vi "Execute Statement.vi"(8 "error in (no error)":errorcluster, 10 "SQL statement":string, 11 "SQLite3LV Cursor in":refnum<class "cursor.lvclass">) -> (0 "error out":errorcluster, 3 "SQLite3LV Cursor out":refnum<class "cursor.lvclass">)   [LabVIEW 2014, in "SQLite3LV.lvlib" / "cursor.lvclass"]
doc: "Executes a single SQL statement. If multiple statements are included in the SQL statement input, only the first statement will be executed.\n\nThe statement may contain unnamed parameters and may return query results.\n\nExamples:\n\nSELECT `LastName` from `Persons`;\n Returns zero or more results of type string. Use \"Column String\" property, followed by the \"Rows Finished?\" property to retrieve results.\n\nSELECT `LastName` from `Persons` WHERE `LastName` GLOB ?\n Returns zero or more results of type string. One string-typed query parameter. Use the \"Bind String\" property node after executing the query to bind the parameter. Use the \"Column String\" and \"Rows Finished?\" property to retrieve results.\n\nSELECT ? + ?;\n Returns a single result of arbitrary type. Accepts two parameters of arbitrary type. Use the \"Bind DBL\" two bind two input parameters. Use the \"Column DBL\" to retrieve the query result."
uses:
  cursor.lvclass
  cursor.lvclass/cursor.ctl
  SQLite3LV.lvlib
  SQLite3 Class/sqlite3.lvclass
  sqlite3_64.dll
panel:
  out "finished?":bool
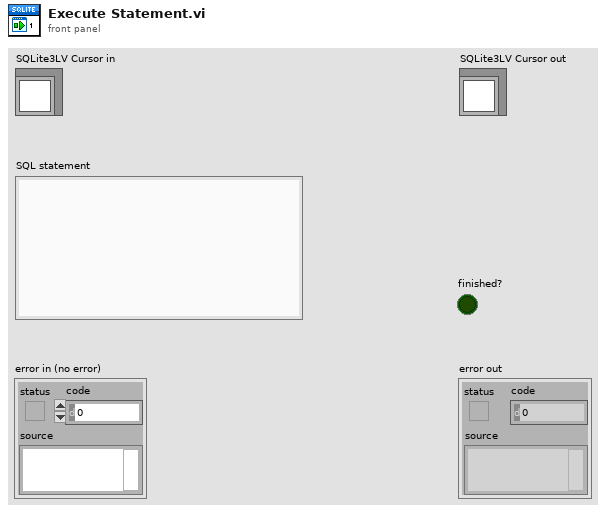
[diagram p1: front panel]
types:
  T1 = typedef "SQLite3LV.lvlib/cursor.lvclass/ctl_active_statement.ctl" = cluster{"ppStmt":i64, "column count":i32, "bind offset":i32, "bind param count":i32, "finished?":bool, "column offset":i32, "column types":i32[]}
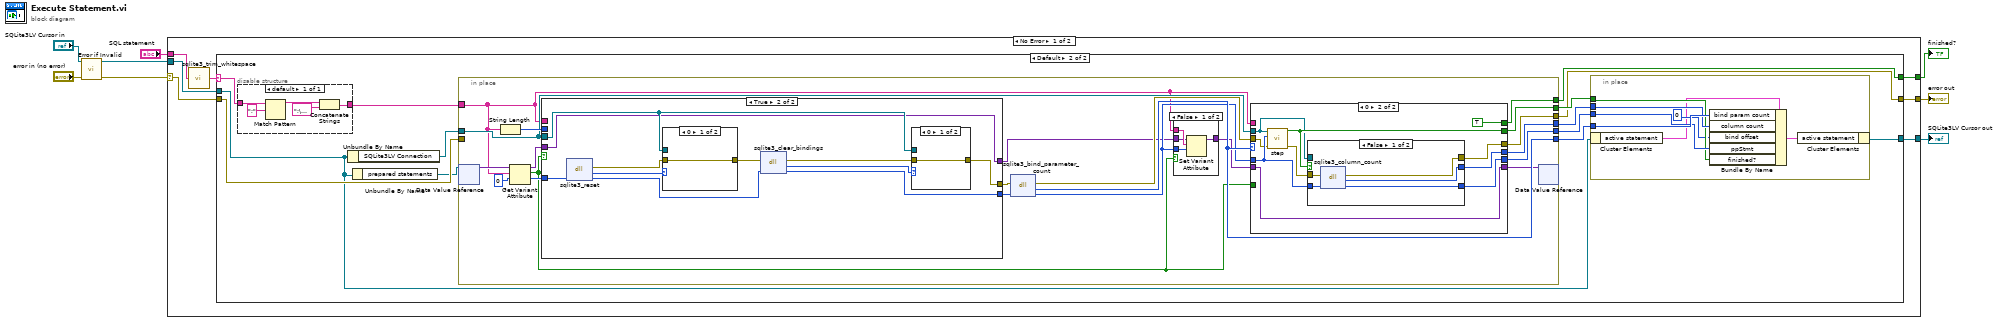
[diagram p0: block diagram]
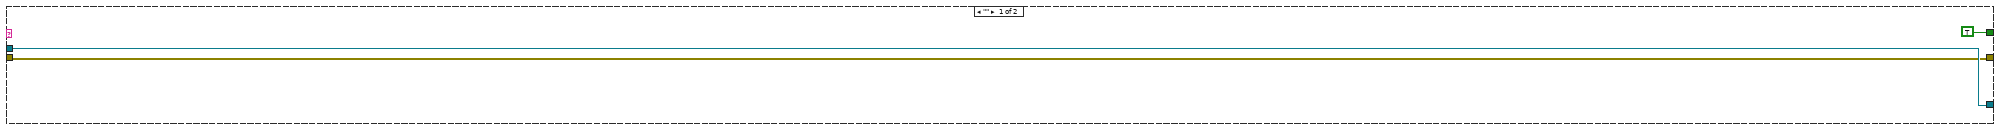
[diagram p2: hidden frame]
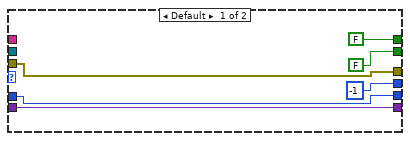
[diagram p4: hidden frame]
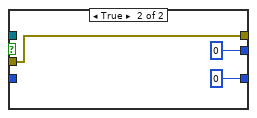
[diagram p5: hidden frame]
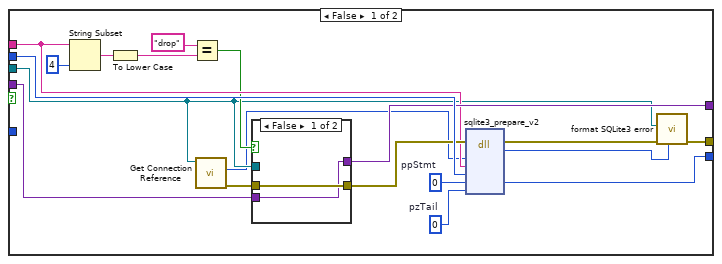
[diagram p6: hidden frame]
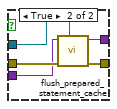
[diagram p7: hidden frame]
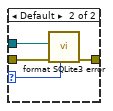
[diagram p8: hidden frame]
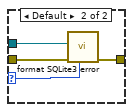
[diagram p9: hidden frame]
diagram:
  n1 = call "Error if Invalid.vi"("error in (no error)"="error in (no error)", "SQLite3LV Cursor in"="SQLite3LV Cursor in") -> ("error out"=w1:errorcluster, "SQLite3LV Cursor out"=w2:refnum<class "cursor.lvclass">)  [unwired: 8 in]
  n2 = case shown="No Error" w1 {
    selector: w1 -> [w10 w142]
    tunnel: [w9 w142] -> w8
    tunnel: [w11 w141] -> w7
    tunnel: w2 -> [w12 w141]
    tunnel: "SQL statement" -> [w15 _]
    tunnel: [w14 _] -> w5
    frame No Error {
      n3 = call "sqlite3_trim_whitespace.vi"("string"=w15) -> ("trimmed string"=w13:string)  [unwired: 1 in]
      n4 = case shown="Default" w13 {
        selector: w13 -> [_ w29]
        tunnel: w12 -> [w17 w19]
        tunnel: [TRUE w31] -> w14
        tunnel: [w17 w22] -> w11
        tunnel: w10 -> [w16 w23]
        tunnel: [w16 w24] -> w9
        frame "" {
        }
        frame Default {
          n5 = disable-structure shown="default" {
            disable-tunnel: [w36] -> w30
            disable-tunnel: w29 -> [w35]
            frame Enabled {
              n6 = Match Pattern(string=w35, regular expression=";") -> (before substring=w32:string)  [unwired: 1 in, 3 out]
              n7 = Concatenate Strings(w32, ";\u0000" ("string")) -> (w36:string)
            }
          }
          n8 = Unbundle By Name(w19) -> ("SQLite3LV Connection"=w20:refnum<class "sqlite3.lvclass">)
          n9 = Unbundle By Name(w19) -> ("prepared statements"=w21:refnum<data-value>)
          n10 = in-place {
            in-place-border: [w55] -> w31
            in-place-border: w30 -> [w39]
            in-place-border: [w52] -> w28
            in-place-border: [w50] -> w27
            in-place-border: [w49] -> w26
            in-place-border: [w48] -> w25
            in-place-border: [w47] -> w24
            in-place-border: w23 -> [_]
            in-place-border: w20 -> [w42]
            n11 = in-place-dvr #1(w21) -> (w45:variant)  [unwired: 1 out]
            n12 = String Length(string=w39) -> (length=w57:i32)
            n13 = Get Variant Attribute(Variant=w45, name=w39, default value (empty Variant)=i64 0) -> (duplicate Variant=w43:variant, found=w41:bool, value=w56:i64)  [unwired: 1 in, 1 out]
            n14 = case shown="True" w41 {
              tunnel: w57 -> [w103 _]
              tunnel: w39 -> [w96 _]
              tunnel: [w101 w116] -> w54
              tunnel: [w100 w120] -> w53
              tunnel: w56 -> [_ w119]
              tunnel: w42 -> [w89 w114]
              tunnel: [w98 w113] -> w38
              tunnel: w43 -> [w90 w113]
              frame False {
                w104 = i64 0  # pzTail
                w105 = i64 0  # ppStmt
                n15 = String Subset(string=w96, length (rest)=4 ("length (rest)")) -> (substring=w94:string)  [unwired: 1 in]
                n16 = To Lower Case(string=w94) -> (all lower case string=w92:string)
                n17 = Equal?(x="drop" ("regular expression"), y=w92) -> (x = y?=w91:bool)
                n18 = call "Get Connection Reference.vi"("SQLite3LV Connection in"=w89) -> ("error out"=w88:errorcluster, "ppDb"=w87:i64)  [unwired: 8 in, 1 out]
                n19 = case shown="False" w91 {
                  tunnel: [w106 w112] -> w98
                  tunnel: [w107 w111] -> w97
                  tunnel: w88 -> [w107 w110]
                  tunnel: w90 -> [w106 w109]
                  tunnel: w89 -> [_ w108]
                  frame False {
                  }
                  frame True {
                    n20 = call "flush_prepared_statement_cache.vi"("SQLite3LV Connection"=w108, "error in (no error)"=w110, "cache in"=w109) -> ("error out"=w111:errorcluster, "cache out"=w112:variant)  [unwired: 7 in]
                  }
                }
                n21 = dll-call lib="C:/Users/BobUser/Desktop/LVTables/sqlite3**.*" fn="sqlite3_prepare_v2"(error in=w97, "pdb"=w87, "zSql"=w96, "nByte"=w103, "ppStmt"=w105, "pzTail"=w104) -> (error out=w99:errorcluster, "result"=w102:i32, "ppStmt"=w100:i64)  [unwired: 6 in, 1 out]
                n22 = call "format SQLite3 error.vi"("SQLite3LV Connection result"=w102, "error in (no error)"=w99, "psqlite"=w89) -> ("error out"=w101:errorcluster)  [unwired: 8 in]
              }
              frame True {
                n23 = dll-call lib="C:/Users/BobUser/Desktop/LVTables/sqlite3**.*" fn="sqlite3_reset"("pStmt"=w119) -> (error out=w122:errorcluster, "result code"=w118:i32, "pStmt"=w123:i64)  [unwired: 3 in, 1 out]
                n24 = case shown="0" w118 {
                  selector: w118 -> [_ w130]
                  tunnel: w122 -> [w129 w133]
                  tunnel: [w129 w132] -> w121
                  tunnel: w114 -> [_ w131]
                  frame 0 {
                  }
                  frame Default {
                    n25 = call "format SQLite3 error.vi"("SQLite3LV Connection result"=w130, "error in (no error)"=w133, "psqlite"=w131) -> ("error out"=w132:errorcluster)  [unwired: 8 in]
                  }
                }
                n26 = dll-call lib="C:/Users/BobUser/Desktop/LVTables/sqlite3**.*" fn="sqlite3_clear_bindings"(error in=w121, "pStmt"=w123) -> (error out=w117:errorcluster, "result code"=w115:i32, "pStmt"=w120:i64)  [unwired: 2 in, 1 out]
                n27 = case shown="0" w115 {
                  selector: w115 -> [_ w126]
                  tunnel: w117 -> [w124 w128]
                  tunnel: [w124 w127] -> w116
                  tunnel: w114 -> [_ w125]
                  frame 0 {
                  }
                  frame Default {
                    n28 = call "format SQLite3 error.vi"("SQLite3LV Connection result"=w126, "error in (no error)"=w128, "psqlite"=w125) -> ("error out"=w127:errorcluster)  [unwired: 8 in]
                  }
                }
              }
            }
            n29 = dll-call lib="C:/Users/BobUser/Desktop/LVTables/sqlite3**.*" fn="sqlite3_bind_parameter_count"(error in=w54, "pStmt"=w53) -> (error out=w51:errorcluster, "count"=w52:i32, "pStmt"=w40:i64)  [unwired: 2 in, 1 out]
            n30 = case shown="False" w41 {
              tunnel: w38 -> [w59 w62]
              tunnel: w39 -> [w61 _]
              tunnel: w40 -> [w60 _]
              tunnel: [w58 w62] -> w37
              frame False {
                n31 = Set Variant Attribute(Variant=w59, name=w61, value=w60) -> (Variant out=w58:variant)  [unwired: 1 in, 2 out]
              }
              frame True {
              }
            }
            n32 = case shown="0" w52 {
              tunnel: w40 -> [w66 w74]
              tunnel: w42 -> [_ w70]
              tunnel: w51 -> [w64 w73]
              tunnel: [FALSE TRUE] -> w55
              tunnel: [-1 ("column count") w77] -> w50
              tunnel: [w66 w76] -> w49
              tunnel: w37 -> [w63 w69]
              tunnel: w41 -> [_ _]
              tunnel: w39 -> [_ _]
              tunnel: [FALSE ("finished?") w72] -> w48
              tunnel: [w64 w71] -> w47
              tunnel: [w63 w69] -> w44
              frame Default {
              }
              frame 0 {
                n33 = call "step.vi"("error in (no error)"=w73, "pStmt"=w74, "psqlite"=w70) -> ("error out"=w75:errorcluster, "finished?"=w72:bool)  [unwired: 7 in]
                n34 = case shown="False" w72 {
                  tunnel: [w83 0 ("column count")] -> w77
                  tunnel: [w82 i64 0 ("pStmt")] -> w76
                  tunnel: w75 -> [w81 w84]
                  tunnel: w74 -> [w80 _]
                  tunnel: [w79 w84] -> w71
                  tunnel: w70 -> [_ _]
                  frame False {
                    n35 = dll-call lib="C:/Users/BobUser/Desktop/LVTables/sqlite3**.*" fn="sqlite3_column_count"(error in=w81, "pStmt"=w80) -> (error out=w79:errorcluster, "column count"=w83:i32, "pStmt"=w82:i64)  [unwired: 2 in, 1 out]
                  }
                  frame True {
                  }
                }
              }
            }
            n36 = in-place-dvr #1(w44) -> ()  [unwired: 2 out]
          }
          n37 = in-place {
            in-place-border: w28 -> [w140]
            in-place-border: w27 -> [w139]
            in-place-border: w26 -> [w138]
            in-place-border: w25 -> [w137]
            n38 = in-place-cluster #2(w19) -> ("active statement"=w134:T1)
            n39 = Bundle By Name(cluster=w134, "bind param count"=w140, "column count"=w139, "bind offset"=0, "ppStmt"=w138, "finished?"=w137) -> (w135:T1)
            n40 = in-place-cluster #2("active statement"=w135) -> (w22:refnum<class "cursor.lvclass">)
          }
        }
      }
    }
    frame Error {
    }
  }
  "error out" <- w8
  "SQLite3LV Cursor out" <- w7
  "finished?" <- w5
